vi "Untitled 15.vi"(8 "error in":errorcluster) -> (0 "error out":errorcluster, 3 "task out":refnum<k21>)   [LabVIEW 2015]
uses:
  <vilib>/DAQmx/create/channels.llb/DAQmx Create Channel (AI-Voltage-Basic).vi
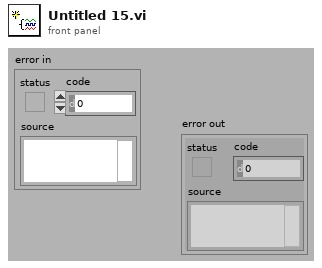
[diagram p1: front panel]
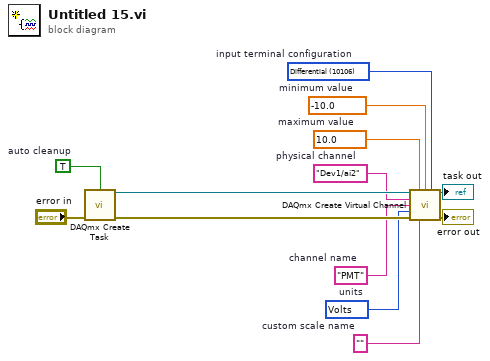
[diagram p0: block diagram]
diagram:
  w1 = 10106 items=["default"=-1, "RSE"=10083, "NRSE"=10078, "Differential"=10106, "Pseudodifferential"=12529]  # input terminal configuration
  w2 = 10348 items=["Volts"=10348, "From Custom Scale"=10065]  # units
  w3 = "PMT"  # channel name
  w6 = ""  # custom scale name
  w7 = -10.0  # minimum value
  w8 = 10.0  # maximum value
  w9 = "Dev1/ai2"  # physical channel
  w11 = TRUE  # auto cleanup
  n1 = call <vilib>:"DAQmx Create Task.vi"("auto cleanup"=w11, "error in"="error in") -> ("task out"=w10:refnum<k21>, "error out"=w12:errorcluster)  [unwired: 12 in]
  n2 = call-poly <vilib>:"DAQmx Create Virtual Channel.vi"("task in"=w10, "maximum value"=w8, "minimum value"=w7, "input terminal configuration"=w1, "physical channels"=w9, "name to assign"=w3, "units"=w2, "error in"=w12, "custom scale name"=w6) -> ("task out"=→"task out":refnum<k21>, "error out"=→"error out":errorcluster)  [unwired: 5 in]
